vi "step_motor_FGV.vi"(7 "Mode":T1, 8 "error in":errorcluster, 11 "Parameter in":variant) -> (0 "error out":errorcluster, 3 "Parameter out":variant)   [LabVIEW 2016]
uses:
  step_motor_modes.ctl
  step_motor_data.ctl
  MainFGV/cluster_main_FGV.ctl
  Config/Channel_config.ctl
  Config/test_config.ctl
  Config/feedType.ctl
  <vilib>/Instr/_visa.llb/VISA Configure Serial Port (Instr).vi
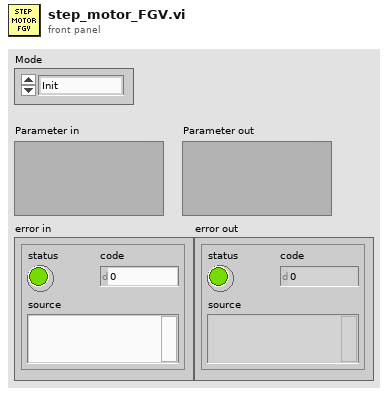
[diagram p1: front panel]
types:
  T1 = typedef "step_motor_modes.ctl" = enum16{"Init", "Config", "OpenCom", "Ajuste", "Step", "End"}
  T2 = typedef "step_motor_data.ctl" = cluster{"SerialPort":refnum<visa-resource-name>, "MinTime":dbl, "baud rate":u32, "data bits":u16, "parity":enum16{"None", "Odd", "Even", "Mark", "Space"}, "stop bits":u16, "flow control":u16, "Steps":i32, "Active":bool}
  T3 = typedef "cluster_main_FGV.ctl" = cluster{"Simulation?":bool, "ChanConfigs":T4[], "Test Config":T5, "Directory":path, "TestName":string, "RawFile":refnum<file>, "InfoFile":refnum<file>, "DataFile":refnum<file>, "task":refnum<k21>, "qRecord":refnum<queue>, "qProcess":refnum<queue>, "feed":T6}
  T4 = typedef "Channel_config.ctl" = cluster{"Canal":i32, "GF":dbl, "SC":bool}
  T5 = typedef "test_config.ctl" = cluster{"HoleDiam":dbl, "MeanLineDiam":dbl, "IncF":dbl, "ElastMod":dbl, "PoissonMod":dbl, "RosType":enum16{"Tipo A", "Tipo B", "Tipo C"}, "Método de análise":enum16{"Não uniforme 2013", "Simplificado 2013", "Simplificado 2008"}, "Pfinal":dbl, "AStop":bool}
  T6 = typedef "feedType.ctl" = enum16{"Manual", "Automático"}
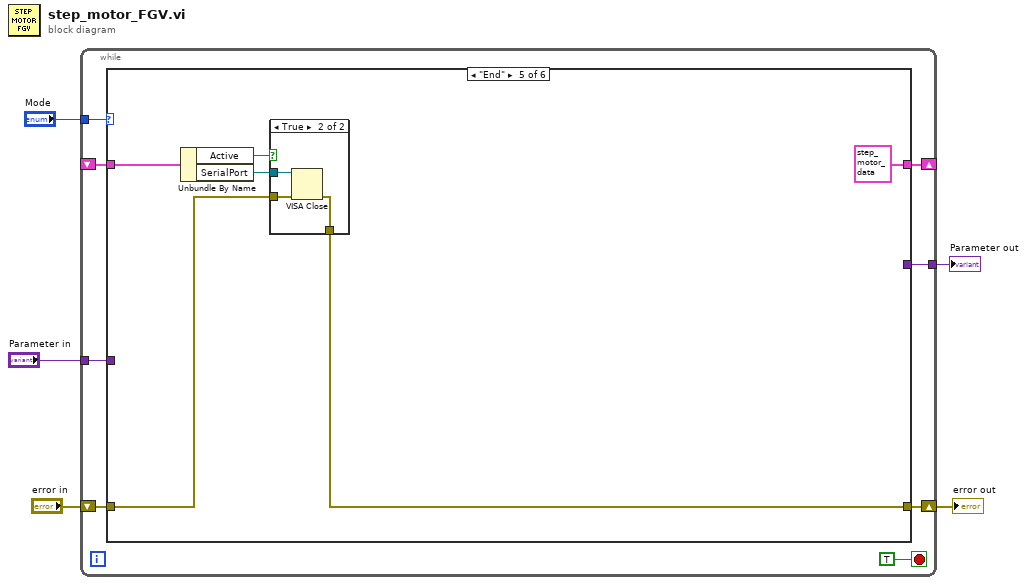
[diagram p0: block diagram]
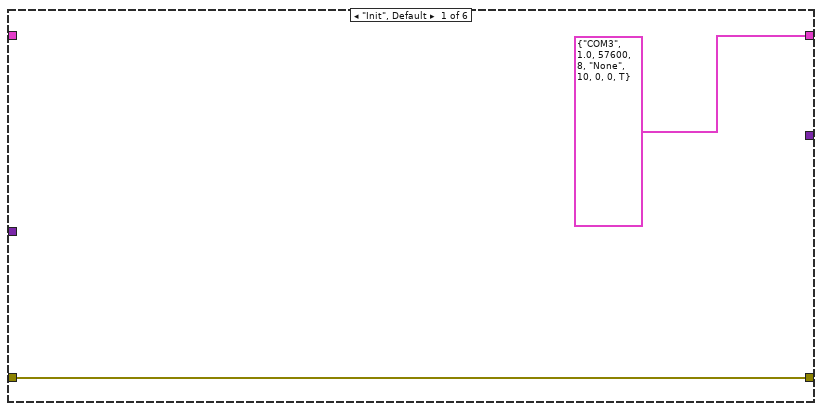
[diagram p2: hidden frame]
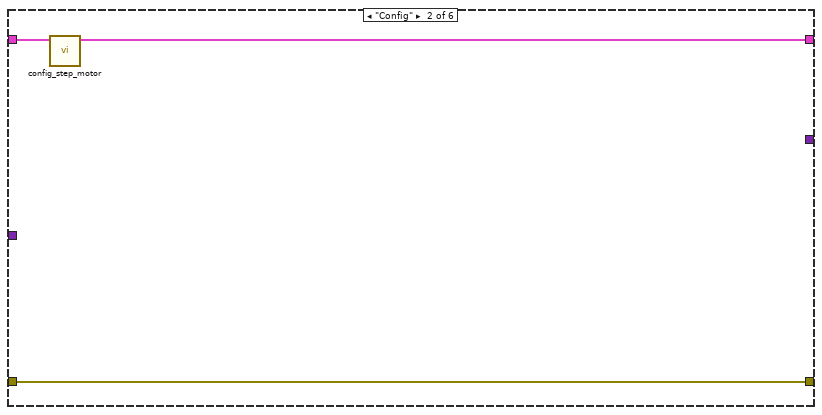
[diagram p3: hidden frame]
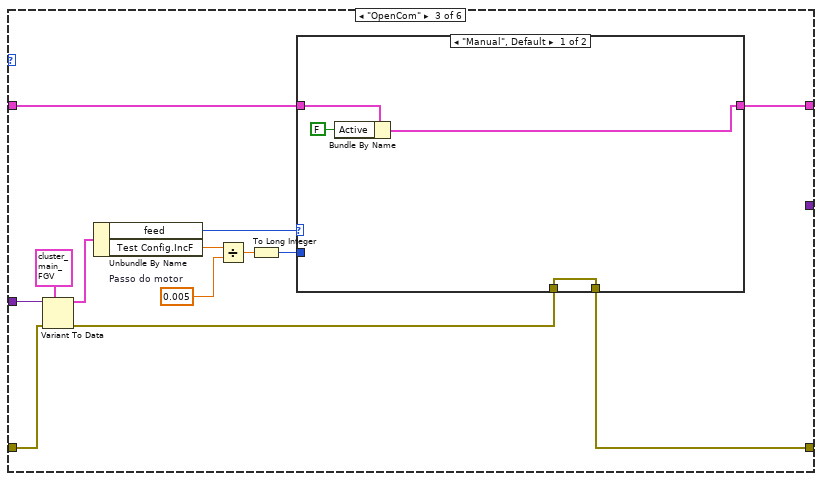
[diagram p4: hidden frame]
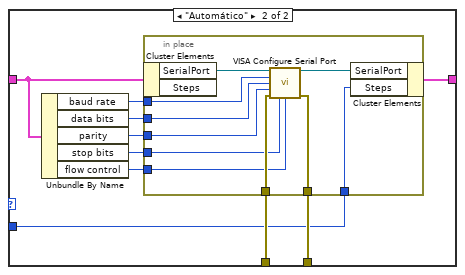
[diagram p5: hidden frame]
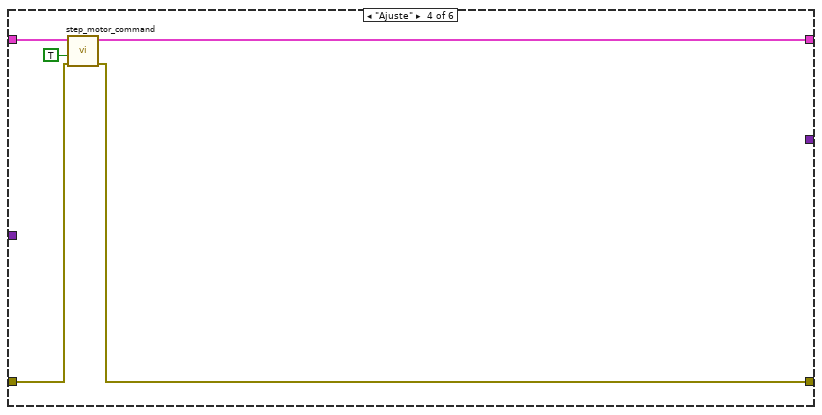
[diagram p6: hidden frame]
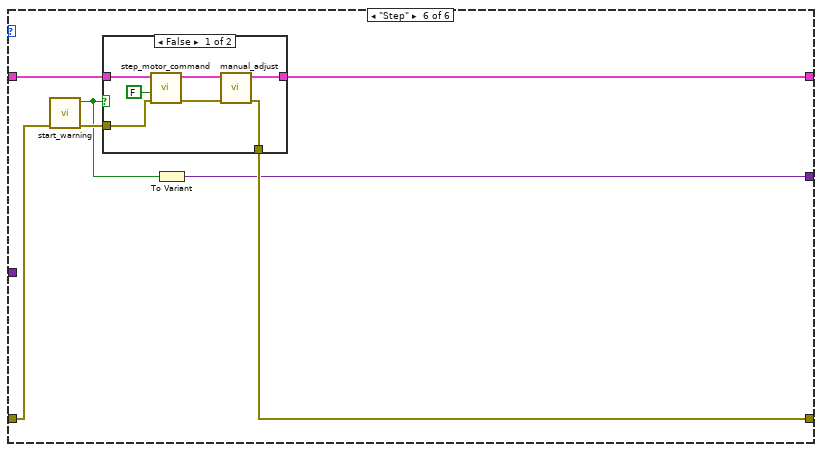
[diagram p8: hidden frame]
diagram:
  n1 = while {
    tunnel: "Mode" -> [w12]
    shift-right: [w11] -> _
    shift-left: _ -> [w10]
    shift-right: [w8] -> w3
    shift-left: "error in" -> [w9]
    tunnel: "Parameter in" -> [w7]
    tunnel: [w6] -> w1
    stop <- TRUE stop-if-true
    n2 = case shown="\"End\"" w12 {
      tunnel: [T2 {"SerialPort"="COM3", "MinTime"=1.0, "baud rate"=57600, "data bits"=8, "parity"=enum."None", "stop bits"=10, "flow control"=0, "Steps"=0, "Active"=TRUE} ("step_motor_data") w17 w30 w59 T2 {"SerialPort"="", "MinTime"=0.0, "baud rate"=57600, "data bits"=8, "parity"=enum."None", "stop bits"=10, "flow control"=0, "Steps"=0, "Active"=FALSE} ("ConfigOut") w75] -> w11
      tunnel: w10 -> [_ w18 w31 w60 w63 w77]
      tunnel: w9 -> [w14 w16 w25 w58 w66 w71]
      tunnel: [w14 w16 w29 w57 w64 w76] -> w8
      tunnel: w7 -> [_ _ w26 _ _ _]
      tunnel: [_ _ _ _ _ w72] -> w6
      frame "Init", Default {
      }
      frame "Config" {
        n3 = call "config_step_motor.vi"("step_motor_data"=w18) -> ("step_motor_data out"=w17:T2)  [unwired: 10 in]
      }
      frame "OpenCom" {
        w22 = 0.005  # Passo do motor
        n4 = Variant To Data(error in=w25, type=T3 {"Simulation?"=FALSE, "ChanConfigs"=[], "Test Config"={"HoleDiam"=1.4, "MeanLineDiam"=5.0, "IncF"=0.2, "ElastMod"=207.0, "PoissonMod"=0.3, "RosType"=enum."Tipo A", "Método de análise"=enum."Simplificado 2008", "Pfinal"=0.3, "AStop"=TRUE}, "Directory"=path "", "TestName"="", "RawFile"=refnum, "InfoFile"=refnum, "DataFile"=refnum, "task"="", "qRecord"=refnum, "qProcess"=refnum, "feed"=enum."Manual"} ("cluster_main_FGV"), Variant=w26) -> (data=w27:T3, error out=w24:errorcluster)
        n5 = Unbundle By Name(w27) -> ("feed"=w19:T6, "Test Config.IncF"=w23:dbl)
        n6 = Divide(x=w23, y=w22) -> (x/y=w21:dbl)
        n7 = To Long Integer(number=w21) -> (32bit integer=w20:i32)
        n8 = case shown="\"Manual\", Default" w19 {
          tunnel: w31 -> [w34 w45]
          tunnel: [w32 w39] -> w30
          tunnel: [w35 w38] -> w29
          tunnel: w24 -> [w35 w37]
          tunnel: w20 -> [_ w36]
          frame "Manual", Default {
            n9 = Bundle By Name(cluster=w34, "Active"=FALSE) -> (w32:T2)
          }
          frame "Automático" {
            n10 = Unbundle By Name(w45) -> ("baud rate"=w44:u32, "data bits"=w43:u16, "parity"=w42:enum16{"None", "Odd", "Even", "Mark", "Space"}, "stop bits"=w41:u16, "flow control"=w40:u16)
            n11 = in-place {
              in-place-border: w37 -> [w55]
              in-place-border: w44 -> [w52]
              in-place-border: w43 -> [w51]
              in-place-border: w42 -> [w50]
              in-place-border: w41 -> [w49]
              in-place-border: w40 -> [w48]
              in-place-border: [w47] -> w38
              in-place-border: w36 -> [w46]
              n12 = in-place-cluster #1(w45) -> ("SerialPort"=w54:refnum<visa-resource-name>)  [unwired: 1 out]
              n13 = call-poly "VISA Configure Serial Port"("VISA resource name"=w54, "baud rate (9600)"=w52, "data bits (8)"=w51, "parity (0:none)"=w50, "error in (no error)"=w55, "stop bits (10: 1 bit)"=w49, "flow control (0:none)"=w48) -> ("VISA resource name out"=w53:refnum<visa-resource-name>, "error out"=w47:errorcluster)  [unwired: 2 in, 5 out]
              n14 = in-place-cluster #1("SerialPort"=w53, "Steps"=w46) -> (w39:T2)
            }
          }
        }
      }
      frame "Ajuste" {
        n15 = call "step_motor_command.vi"("error in"=w58, "Ajuste?"=TRUE, "step_motor_data"=w60) -> ("error out"=w57:errorcluster, "output cluster"=w59:T2)  [unwired: 6 in, 1 out]
      }
      frame "End" {
        n16 = Unbundle By Name(w63) -> ("Active"=w61:bool, "SerialPort"=w62:refnum<visa-resource-name>)
        n17 = case shown="True" w61 {
          tunnel: w66 -> [w67 w70]
          tunnel: [w67 w69] -> w64
          tunnel: w62 -> [_ w68]
          frame False {
          }
          frame True {
            n18 = VISA Close(VISA resource name=w68, error in (no error)=w70) -> (error out=w69:errorcluster)
          }
        }
      }
      frame "Step" {
        n19 = call "start_warning.vi"("error in"=w71) -> ("error out"=w74:errorcluster, "Cancelado?"=w73:bool)  [unwired: 9 in]
        n20 = case shown="False" w73 {
          tunnel: w77 -> [w83 w85]
          tunnel: [w80 w86] -> w76
          tunnel: [w79 w85] -> w75
          tunnel: w74 -> [w78 w86]
          frame False {
            n21 = call "step_motor_command.vi"("error in"=w78, "Ajuste?"=FALSE, "step_motor_data"=w83) -> ("error out"=w82:errorcluster, "output cluster"=w81:T2)  [unwired: 6 in, 1 out]
            n22 = call "manual_adjust.vi"("error in"=w82, "ConfigIn"=w81) -> ("error out"=w80:errorcluster, "ConfigOut"=w79:T2)  [unwired: 8 in]
          }
          frame True {
          }
        }
        n23 = To Variant(anything=w73) -> (Variant=w72:variant)
      }
    }
  }
  "error out" <- w3
  "Parameter out" <- w1
